vi "DesyncInitCAN.vi"(2 "Desync Time (ms)":u32, 3 "error in":errorcluster) -> (1 "error out":errorcluster)   [LabVIEW 2020]
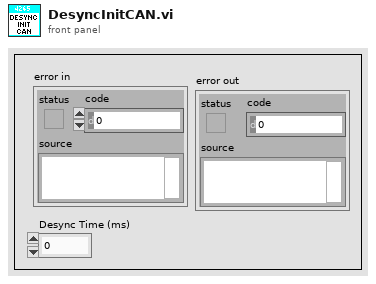
[diagram p1: front panel]
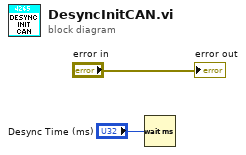
[diagram p0: block diagram]
diagram:
  n1 = Wait (ms)(milliseconds to wait="Desync Time (ms)") -> ()  [unwired: 1 out]
  "error out" <- "error in"
